vi "rapidOX_O2_sensor_subVI.vi"(10 "rapid ox info in":T2) -> (2 "rapidox info out":T1)   [LabVIEW 2014]
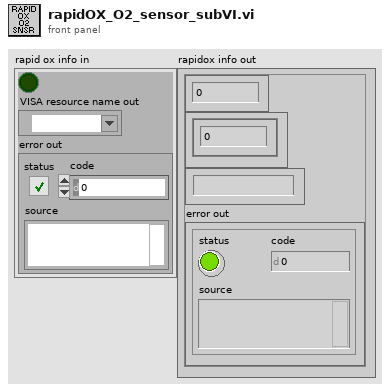
[diagram p1: front panel]
types:
  T1 = cluster{"Numeric Control":dbl, "Cluster":cluster{"Numeric Control":dbl}, "String":string, "error out":errorcluster}
  T2 = cluster{bool, "VISA resource name out":refnum<visa-resource-name>, "error out":errorcluster}
  T3 = cluster{dbl, cluster{dbl}, string, "error out":errorcluster}
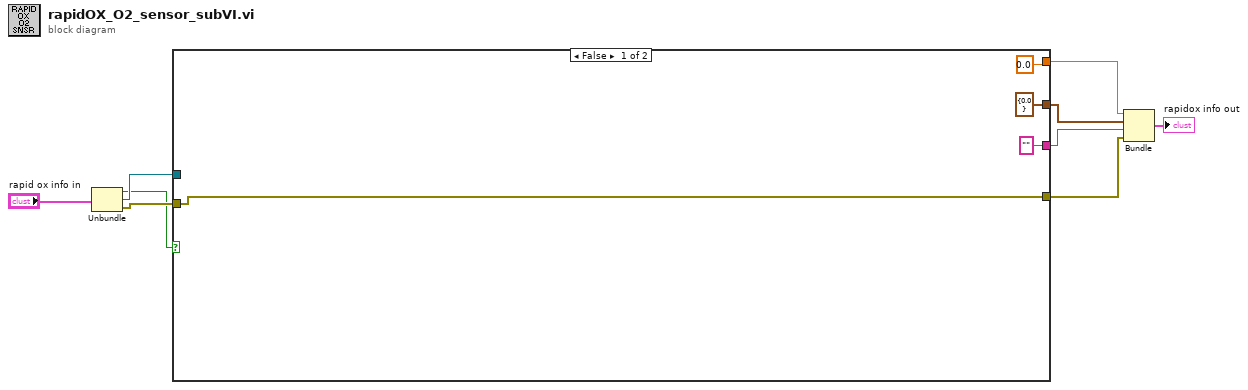
[diagram p0: block diagram]
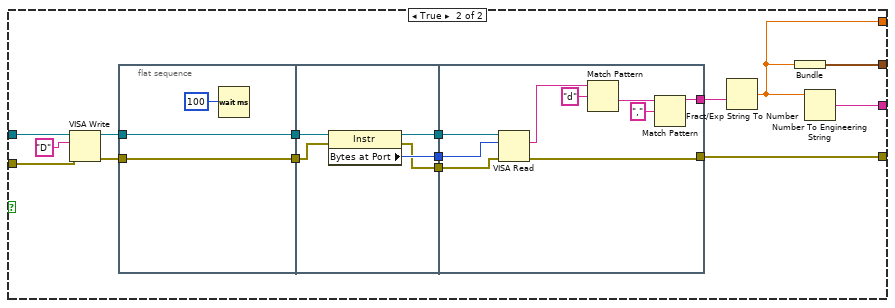
[diagram p2: hidden frame]
diagram:
  n1 = Unbundle("rapid ox info in") -> (w6:bool, "VISA resource name out"=w7:refnum<visa-resource-name>, "error out"=w8:errorcluster)
  n2 = case shown="False" w6 {
    tunnel: [cluster{dbl} {0.0} w23] -> w4
    tunnel: [0.0 w22] -> w5
    tunnel: [w10 w21] -> w2
    tunnel: ["" w19] -> w3
    tunnel: w8 -> [w10 w18]
    tunnel: w7 -> [_ w17]
    frame False {
    }
    frame True {
      n3 = VISA Write(VISA resource name=w17, write buffer="D", error in (no error)=w18) -> (VISA resource name out=w15:refnum<visa-resource-name>, error out=w16:errorcluster)  [unwired: 1 out]
      n4 = flat-sequence {
        tunnel: [w31] -> w28
        tunnel: [w29] -> w27
        tunnel: w15 -> [w31]
        tunnel: w16 -> [w29]
        tunnel: w28 -> [w36]
        tunnel: w27 -> [w35]
        tunnel: [w34] -> w26
        tunnel: [w33] -> w25
        tunnel: [w32] -> w24
        tunnel: w26 -> [w45]
        tunnel: w25 -> [w44]
        tunnel: w24 -> [w43]
        tunnel: [w42] -> w21
        tunnel: [w37] -> w20
        frame #0 {
          n5 = Wait (ms)(milliseconds to wait=u32 100) -> ()  [unwired: 1 out]
        }
        frame #1 {
          n6 = property class="Instr"(reference=w36, error in=w35) -> (reference out=w34:refnum<visa-resource-name>, error out=w32:errorcluster, "Bytes at Port"=w33:u32)
        }
        frame #2 {
          n7 = VISA Read(VISA resource name=w45, byte count=w44, error in (no error)=w43) -> (read buffer=w40:string, error out=w42:errorcluster)  [unwired: 2 out]
          n8 = Match Pattern(string=w40, regular expression="d") -> (after substring=w38:string)  [unwired: 1 in, 3 out]
          n9 = Match Pattern(string=w38, regular expression=",") -> (before substring=w37:string)  [unwired: 1 in, 3 out]
        }
      }
      n10 = Fract/Exp String To Number(string=w20) -> (number=w22:dbl)  [unwired: 3 in, 1 out]
      n11 = Bundle(w22) -> (w23:cluster{dbl})  [unwired: 1 in]
      n12 = Number To Engineering String(4:w22) -> (0:w19:string)  [unwired: 3 in]
    }
  }
  n13 = Bundle(w5, w4, w3, "error out"=w2) -> (→"rapidox info out":T3)  [unwired: 1 in]
